vi "PH_SSAC.set modified data.vi"(0 "i ref in":refnum<vi>, 2 "i attribute":T1={"GUI Refs"={"Delete"=refnum, "Global On"=refnum, "Cam Source"=refnum, "Frame Main Signal"=refnum, "Frame Background"=refnum, "dt (Gauss smooth)"=refnum, "Calibration Factor"=refnum, "Background acquire"=refnum, "Threshold"=refnum, "Time evolution of mean pulse duration"=refnum, "Mean Pulse Duration"=refnum, "Main signal"=refnum, "Current Pulse Duration"=refnum, "Processed"=refnum, "Saturation"=refnum, "# for Average"=refnum, "Position"=refnum, "BG Status"=refnum, "Save BG data"=refnum, "Read BG Data"=refnum, "Background Calibration Data"=refnum}, "Images"={"OP Image"=refnum, "GUI Image"=refnum, "PSDB Image"=refnum}, "Global On?"=FALSE, "Frame Main"={"x"=0, "dx"=1280, "y"=150, "dy"=150}, "Frame Background"={"x"=0, "dx"=100, "y"=400, "dy"=250}, "dt [fs]"=1.0, "Calibration Factor [fs/pixel]"=1.0, "Threshold"=0.0, "Time evolution of mean pulse duration [fs]"=[], "Main Signal"={"Time for Main"=[], "Signal"=[]}, "Processed"=FALSE, "Current Pulse Duration [fs]"=0.0, "# for Average"=1, "Position"=0, "Pulse Durations [fs]"=[], "BG"={"Acquire?"=FALSE, "Background Calibration Data"={"Date"="", "Time"="", "Frame Main"={"x"=0, "dx"=0, "y"=0, "dy"=0}, "dt [fs]"=0.0, "Calibration Factor [fs/pixel]"=0.0, "Signal"=array[1280 elements], "Frame Background"={"x"=0, "dx"=100, "y"=400, "dy"=250}}, "Save Data"=FALSE}}, 5 "error in (no error)":errorcluster) -> (14 "i ref out":refnum<vi>, 19 "error out":errorcluster)   [LabVIEW 2014, in "PH_SSAC.lvlib"]
doc: "Writes the data into the attribute of an object. Then, the attribute dara are unlocked using the \"release\" method. Prior to calling THIS method, the attribute data must have been locked using the methods \"lock\" or \"get data to modify\".\n\n\nLicense Agreement for this software:\n\nCopyright (C)\nGesellschaft für Schwerionenforschung, GSI\nPlanckstr. 1\n64291 Darmstadt\nGermany\n\nContact: D.Beck@gsi.de \n\nThis program is free software; you can redistribute it and/or modify it under the terms of the GNU General Public License as published by the Free Software Foundation; either version 2 of the license, or (at your option) any later version.\n\nThis program is distributed in the hope that it will be useful, but WITHOUT ANY WARRANTY; without even the implied warranty of MERCHANTABILITY or FITNESS FOR A PARTICULAR PURPOSE. See the GNU General License for more details (http://www.gnu.org).\n\nGesellschaft für Schwerionenforschung, GSI\nPlanckstr. 1, 64291 Darmstadt, Germany\nFor all questions and ideas contact: M.Richter@gsi.de, H.Brand@gsi.de or D.Beck@gsi.de.\nLast update: 17-JUN-2004"
uses:
  PH_SSAC.lvlib
  PH_SSAC.i attribute.ctl
  <vilib>/vision/Image Controls.llb/IMAQ Image.ctl
  PH_SSAC.Background Data.ctl
  CSCore/CSObj/CSObj.lvlib
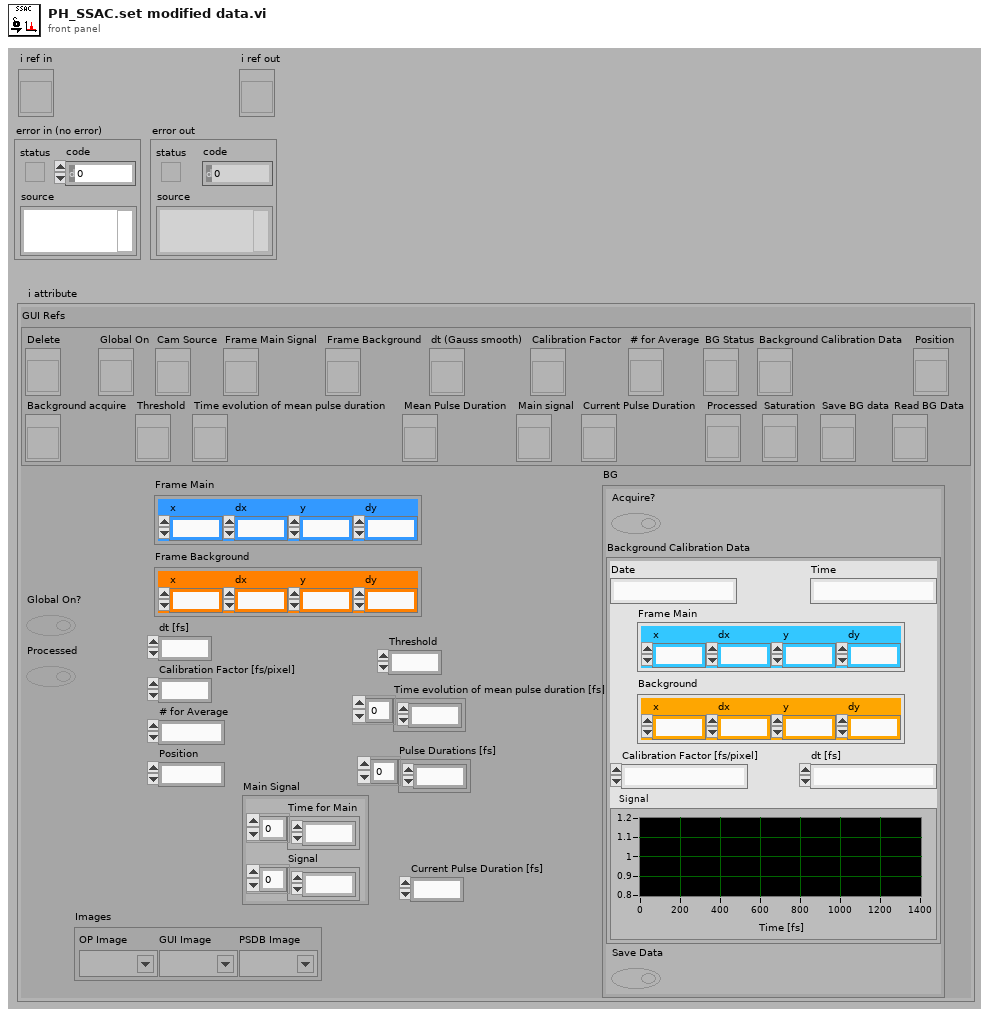
[diagram p1: front panel]
types:
  T1 = typedef "PH_SSAC.lvlib/PH_SSAC.i attribute.ctl" = cluster{"GUI Refs":cluster{"Delete":refnum<vi>, "Global On":refnum<vi>, "Cam Source":refnum<vi>, "Frame Main Signal":refnum<vi>, "Frame Background":refnum<vi>, "dt (Gauss smooth)":refnum<vi>, "Calibration Factor":refnum<vi>, "Background acquire":refnum<vi>, "Threshold":refnum<vi>, "Time evolution of mean pulse duration":refnum<vi>, "Mean Pulse Duration":refnum<vi>, "Main signal":refnum<vi>, "Current Pulse Duration":refnum<vi>, "Processed":refnum<vi>, "Saturation":refnum<vi>, "# for Average":refnum<vi>, "Position":refnum<vi>, "BG Status":refnum<vi>, "Save BG data":refnum<vi>, "Read BG Data":refnum<vi>, "Background Calibration Data":refnum<vi>}, "Images":cluster{"OP Image":T2, "GUI Image":T2, "PSDB Image":T2}, "Global On?":bool, "Frame Main":cluster{"x":u32, "dx":u32, "y":u32, "dy":u32}, "Frame Background":cluster{"x":u32, "dx":u32, "y":u32, "dy":u32}, "dt [fs]":dbl, "Calibration Factor [fs/pixel]":dbl, "Threshold":dbl, "Time evolution of mean pulse duration [fs]":dbl[], "Main Signal":cluster{"Time for Main":dbl[], "Signal":dbl[]}, "Processed":bool, "Current Pulse Duration [fs]":dbl, "# for Average":i32, "Position":i32, "Pulse Durations [fs]":dbl[], "BG":cluster{"Acquire?":bool, "Background Calibration Data":T3, "Save Data":bool}}
  T2 = typedef "IMAQ Image.ctl" = refnum<image>
  T3 = typedef "PH_SSAC.lvlib/PH_SSAC.Background Data.ctl" = cluster{"Date":string, "Time":string, "Frame Main":cluster{"x":u32, "dx":u32, "y":u32, "dy":u32}, "dt [fs]":dbl, "Calibration Factor [fs/pixel]":dbl, "Signal":dbl[], "Frame Background":cluster{"x":u32, "dx":u32, "y":u32, "dy":u32}}
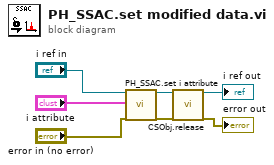
[diagram p0: block diagram]
diagram:
  n1 = call "PH_SSAC.set i attribute.vi"("i ref in"="i ref in", "i attribute"="i attribute", "error in (no error)"="error in (no error)") -> ("i ref out"=w4:refnum<vi>, "error out"=w3:errorcluster)  [unwired: 15 in]
  n2 = call "CSObj.release.vi"("i ref in"=w4, "error in (no error)"=w3) -> ("i ref out"=→"i ref out":refnum<vi>, "error out"=→"error out":errorcluster)  [unwired: 16 in]
